vi "Check Folder Path.vi"(8 "error in":errorcluster, 11 "Path In":path) -> (0 "error out":errorcluster, 3 "Path Out":path)   [LabVIEW 2017]
uses:
  <vilib>/Utility/sysdir.llb/System Directory Type.ctl
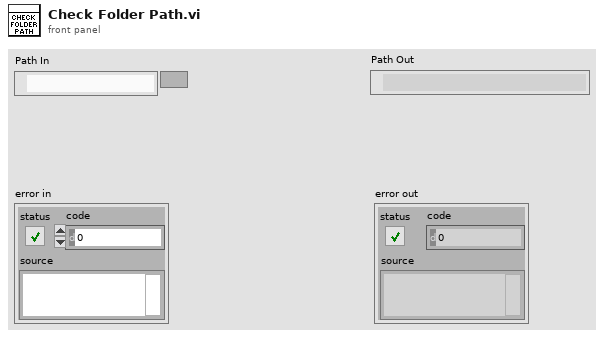
[diagram p1: front panel]
types:
  T1 = typedef "System Directory Type.ctl" = i32
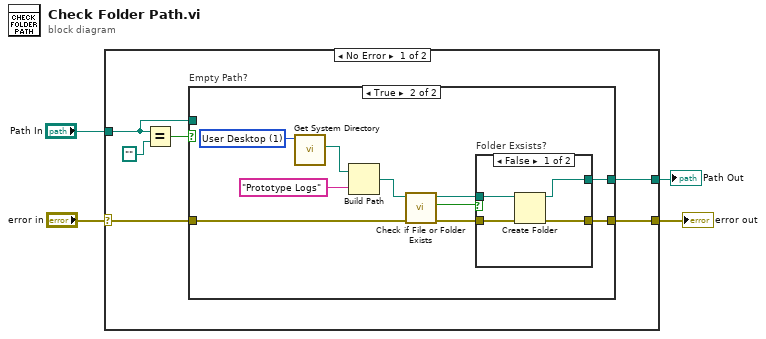
[diagram p0: block diagram]
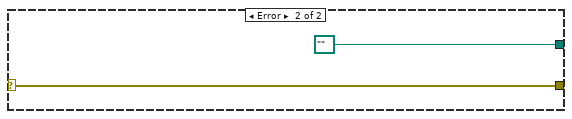
[diagram p4: hidden frame]
diagram:
  n1 = case shown="No Error" "error in" {
    selector: "error in" -> [w6 w30]
    tunnel: "Path In" -> [w7 _]
    tunnel: [w8 path "" ("appended path")] -> w2
    tunnel: [w5 w30] -> w1
    frame No Error {
      n2 = Equal?(x=w7, y=path "") -> (x = y?=w9:bool)
      n3 = case "Empty Path?" shown="True" w9 {
        tunnel: [w12 w13] -> w8
        tunnel: w7 -> [w12 _]
        tunnel: w6 -> [w11 w15]
        tunnel: [w11 w14] -> w5
        frame False {
        }
        frame True {
          w22 = T1 1 items=["User Home"=0, "User Desktop"=1, "User Documents"=2, "User Application Data"=3, "User Preferences"=4, "User Temporary"=5, "Public Documents"=6, "Public Application Data"=7, "Public Preferences"=8, "Public Cache"=13, "System Core Libraries"=9, "System Installed Libraries"=10, "Application Files"=11, "Boot Volume Root"=12] ("system directory type")
          n4 = call <vilib>:"Get System Directory.vi"("system directory type"=w22) -> ("system directory"=w21:path)  [unwired: 10 in]
          n5 = Build Path(base path=w21, name or relative path="Prototype Logs") -> (appended path=w19:path)
          n6 = call <vilib>:"Check if File or Folder Exists.vi"("error in (no error)"=w15, "path"=w19) -> ("error out"=w16:errorcluster, "file or folder exists?"=w18:bool, "dup path"=w17:path)  [unwired: 7 in]
          n7 = case "Folder Exsists?" shown="False" w18 {
            tunnel: w17 -> [w26 w27]
            tunnel: w16 -> [w25 w28]
            tunnel: [w24 w28] -> w14
            tunnel: [w23 w27] -> w13
            frame False {
              n8 = Create Folder(path (use dialog)=w26, error in=w25) -> (created path=w23:path, error out=w24:errorcluster)  [unwired: 1 in, 1 out]
            }
            frame True {
            }
          }
        }
      }
    }
    frame Error {
    }
  }
  "error out" <- w1
  "Path Out" <- w2
